vi "Load Settings from XML.vi"(8 "error in (no error)":errorcluster caption="错误输入（无错误）", 11 "名称或相对路径":string) -> (0 "error out":errorcluster caption="错误输出", 2 "XML Elements":string caption="XML元素")   [LabVIEW 2015]
doc: "尝试从XML文件加载先前的用户设置。\n\n该VI不会生成错误。如无法加载和解析XML文件，直接返回默认设置。"
uses:
  <vilib>/Utility/xml.llb/Read From XML File(string).vi
panel:
  # "（向上滚动可查看设置控件）"
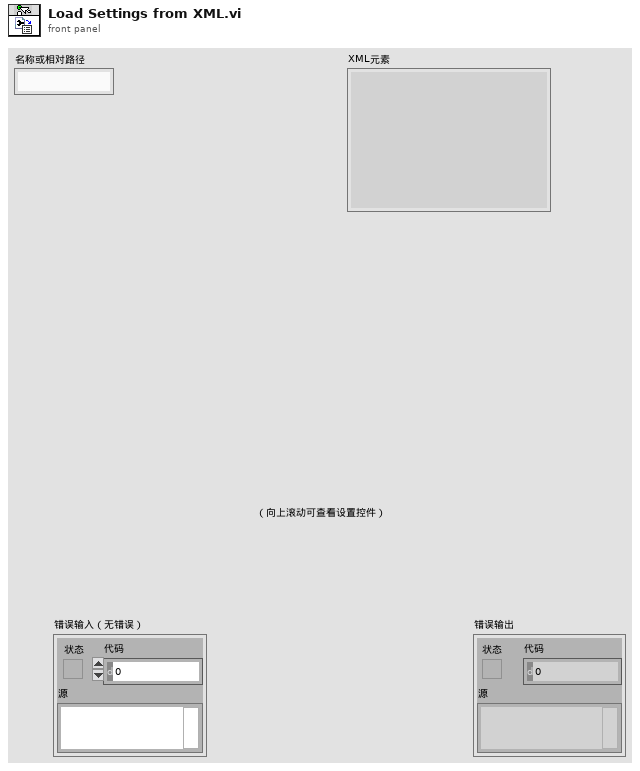
[diagram p1: front panel]
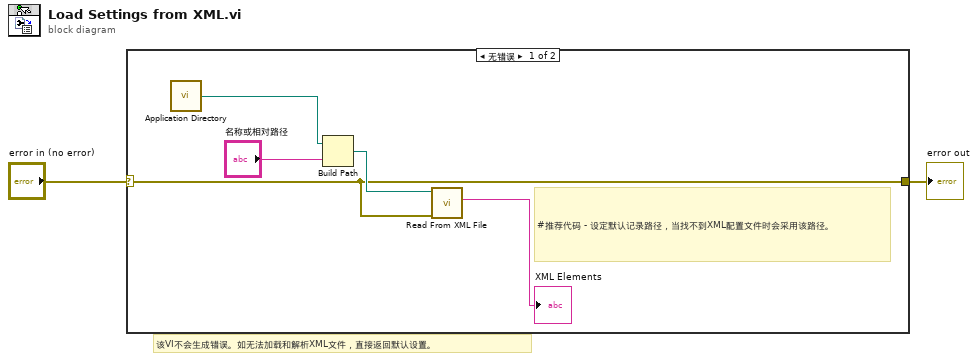
[diagram p0: block diagram]
diagram:
  # "该VI不会生成错误。如无法加载和解析XML文件，直接返回默认设置。"
  n1 = case shown="无错误" "error in (no error)" {
    selector: "error in (no error)" -> [w4 w8]
    tunnel: [w4 w8] -> w1
    frame No Error {
      # "#推荐代码 - 设定默认记录路径，当找不到XML配置文件时会采用该路径。"
      n2 = call <vilib>:"Application Directory.vi"() -> ("Application Directory"=w7:path)
      n3 = Build Path(base path=w7, name or relative path="名称或相对路径") -> (appended path=w6:path)
      n4 = call-poly <vilib>:"Read From XML File.vi"("error in (no error)"=w4, "XML File Path"=w6) -> ("XML Elements"=→"XML Elements":string)  [unwired: 7 in, 2 out]
    }
    frame Error {
    }
  }
  "error out" <- w1
